vi "Configure Lockout.vi"(0 "VISA resource name":refnum<visa-resource-name>, 1 "Lock Dispense Time":bool, 2 "Lock Dispense Mode":bool, 3 "Lock Dispense Pressure":bool, 4 "Lock Deposit Counter":bool, 5 "Lock Main Menu":bool, 6 "Lock AI Mode":bool, 7 "error in (no error)":errorcluster, 8 "Lock Memory Cell Selection":bool, 9 "Lock Alarm Options":bool, 10 "Lock Dispense Vacuum":bool, 11 "Lock Alarms Reset":bool, 12 "Password (0000)":i32 format="%04.0f", 13 "Lock AI Reset":bool) -> (20 "VISA resource name out":refnum<visa-resource-name>, 27 "error out":errorcluster)   [LabVIEW 2018, in "EFD Ultimus V.lvlib"]
doc: "Updates the operator lockout settings. A '1' indicates that a feature is locked out. A '0' indicates that the feature is not locked out.\nHost Format:\nEG--PAppppDTtDPpDVvMmDCcDMdAIaARuALbMMePUfVUgLAhCLjCOkAMn\n\npppp: Four digit password. This needs to match the password set on the dispenser. The dispenser will return an error if incorrect.\nt: lock out dispense time: '1'=lockout, '0'=enabled\np: lockout dispense pressure: \nv: lockout dispense vacuum: \nm: lockout memory cell selection: \nc: lockout deposit counter selection:\nd: lockout dispense mode change: \na: lockout Auto Increment Mode selection: \nu: lockout Auto Increment Reset:\nb: lockout Alarms Reset:\ne: lockout Main Menu selection: \nf: lockout Pressure Unit Menu selection: \ng: lockout Vacuum Unit Menu selection: \nh: lockout Language Menu selection: \nj: lockout Set Clock/Date Menu selection: \nk: lockout Set Communications Menu selection: \nn: lockout Alarm Options Menu selection:"
uses:
  EFD Ultimus V.lvlib
panel:
  # "NOTE: Communications,Clock/Date,Vacuum Unit, Pressure Unit and Language Selection are defaulted to enabled.\nConsider locking out the main menu, to prohibit these operations if needed."
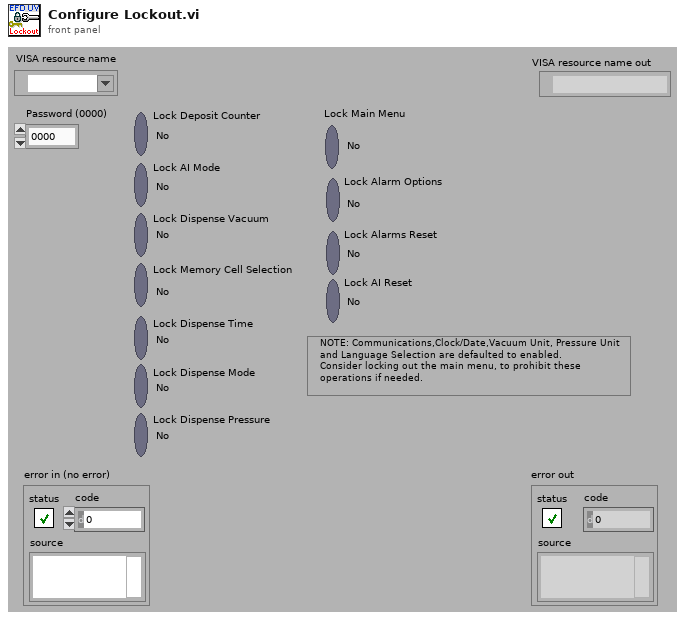
[diagram p1: front panel]
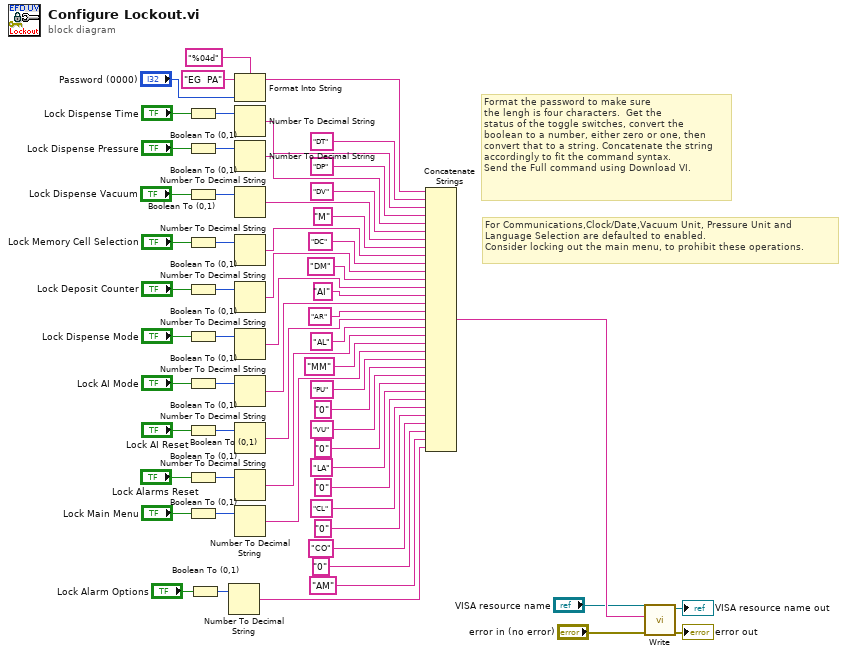
[diagram p0: block diagram]
diagram:
  # "For Communications,Clock/Date,Vacuum Unit, Pressure Unit and \nLanguage Selection are defaulted to enabled.\nConsider locking out the main menu, to prohibit these operations."
  # "Format the password to make sure\nthe lengh is four characters.  Get the \nstatus of the toggle switches, convert the \nboolean to a number, either zero or one, then\nconvert that to a string. Concatenate the string\naccordingly to fit the command syntax. \nSend the Full command using Download VI."
  n1 = Boolean To (0,1)(Boolean="Lock Dispense Time") -> (0, 1=w32:i16)
  n2 = Boolean To (0,1)(Boolean="Lock Dispense Pressure") -> (0, 1=w34:i16)
  n3 = Boolean To (0,1)(Boolean="Lock Dispense Vacuum") -> (0, 1=w37:i16)
  n4 = Boolean To (0,1)(Boolean="Lock Memory Cell Selection") -> (0, 1=w40:i16)
  n5 = Boolean To (0,1)(Boolean="Lock Deposit Counter") -> (0, 1=w43:i16)
  n6 = Boolean To (0,1)(Boolean="Lock Dispense Mode") -> (0, 1=w46:i16)
  n7 = Boolean To (0,1)(Boolean="Lock AI Mode") -> (0, 1=w49:i16)
  n8 = Boolean To (0,1)(Boolean="Lock AI Reset") -> (0, 1=w52:i16)
  n9 = Boolean To (0,1)(Boolean="Lock Alarms Reset") -> (0, 1=w55:i16)
  n10 = Boolean To (0,1)(Boolean="Lock Main Menu") -> (0, 1=w58:i16)
  n11 = Boolean To (0,1)(Boolean="Lock Alarm Options") -> (0, 1=w62:i16)
  n12 = Number To Decimal String(number=w62) -> (decimal integer string=w63:string)  [unwired: 1 out]
  n13 = Format Into String(format string="%04d", initial string="EG  PA" ("Command To Write"), "Password (0000)") -> (resulting string=w6:string)  [unwired: 1 in, 1 out]
  n14 = Number To Decimal String(number=w32) -> (decimal integer string=w33:string)  [unwired: 1 out]
  n15 = Number To Decimal String(number=w34) -> (decimal integer string=w36:string)  [unwired: 1 out]
  n16 = Number To Decimal String(number=w37) -> (decimal integer string=w39:string)  [unwired: 1 out]
  n17 = Number To Decimal String(number=w40) -> (decimal integer string=w42:string)  [unwired: 1 out]
  n18 = Number To Decimal String(number=w43) -> (decimal integer string=w45:string)  [unwired: 1 out]
  n19 = Number To Decimal String(number=w46) -> (decimal integer string=w48:string)  [unwired: 1 out]
  n20 = Number To Decimal String(number=w49) -> (decimal integer string=w51:string)  [unwired: 1 out]
  n21 = Number To Decimal String(number=w52) -> (decimal integer string=w54:string)  [unwired: 1 out]
  n22 = Number To Decimal String(number=w55) -> (decimal integer string=w57:string)  [unwired: 1 out]
  n23 = Number To Decimal String(number=w58) -> (decimal integer string=w60:string)  [unwired: 1 out]
  n24 = Concatenate Strings(w6, "DT" ("string"), w33, "DP" ("string"), w36, "DV" ("string"), w39, "M" ("string"), w42, "DC" ("string"), w45, "DM" ("string"), w48, "AI" ("string"), w51, "AR" ("string"), w54, "AL" ("string"), w57, "MM" ("string"), w60, "PU" ("string"), "0" ("string"), "VU" ("string"), "0" ("string"), "LA" ("string"), "0" ("string"), "CL" ("string"), "0" ("string"), "CO" ("string"), "0" ("string"), "AM" ("string"), w63) -> (w14:string)
  n25 = call "Write.vi"("error in (no error)"="error in (no error)", "Command To Write"=w14, "VISA resource name"="VISA resource name") -> ("error out"=→"error out":errorcluster, "VISA resource name out"=→"VISA resource name out":refnum<visa-resource-name>)  [unwired: 7 out]
